vi "PROTECAO_AH.vi"(11 "AH_Destino":dbl format="%.9g") -> (3 "CONT AH":i32)   [LabVIEW 2018]
uses:
  Global_Telescopio.vi
panel:
  out "DIST AH":dbl
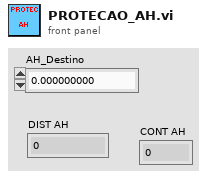
[diagram p1: front panel]
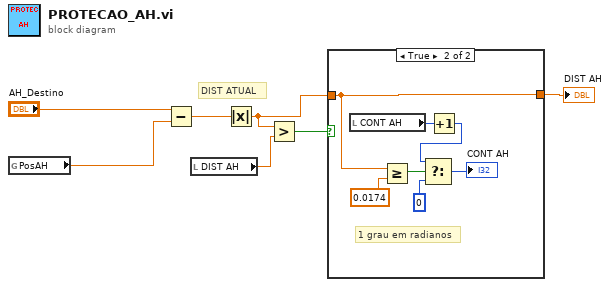
[diagram p0: block diagram]
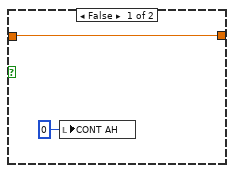
[diagram p2: hidden frame]
diagram:
  # "DIST ATUAL"
  n1 = global read "Global_Telescopio.vi" "PosAH"() -> (w7:dbl)
  n2 = Subtract(x="AH_Destino", y=w7) -> (x-y=w6:dbl)
  n3 = local read "DIST AH"() -> (w5:dbl)
  n4 = Absolute Value(x=w6) -> (abs(x)=w2:dbl)
  n5 = Greater?(x=w2, y=w5) -> (0:w4:bool)
  n6 = case shown="True" w4 {
    tunnel: w2 -> [w9 w13]
    tunnel: [w9 w13] -> w3
    frame False {
      n7 = local write "CONT AH"(0 ("CONT AH")) -> ()
    }
    frame True {
      # "1 grau em radianos"
      n8 = local read "CONT AH"() -> (w11:i32)
      n9 = Greater Or Equal?(x=w13, y=0.0174) -> (x >= y?=w15:bool)
      n10 = Increment(x=w11) -> (x+1=w10:i32)
      n11 = Select(t=w10, s=w15, f=0 ("t")) -> (s? t:f=→"CONT AH":i32)
    }
  }
  "DIST AH" <- w3
